vi "Has Run Once.vi"(8 "error in (no error)":errorcluster, 11 "CommandDirector in":refnum<class "CommandDirector.lvclass">) -> (0 "error out":errorcluster, 2 "Has Run Once":bool, 3 "CommandDirector out":refnum<class "CommandDirector.lvclass">)   [LabVIEW 2023, in "HAF.lvlib" / "CommandDirector.lvclass"]
uses:
  CommandDirector.lvclass
  CommandDirector.lvclass/CommandDirector.ctl
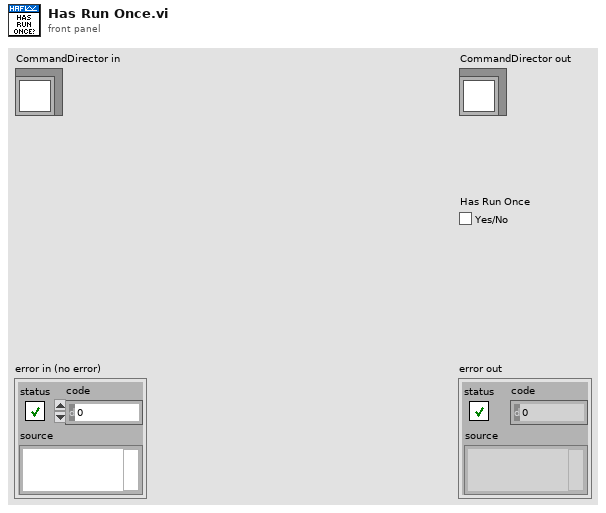
[diagram p1: front panel]
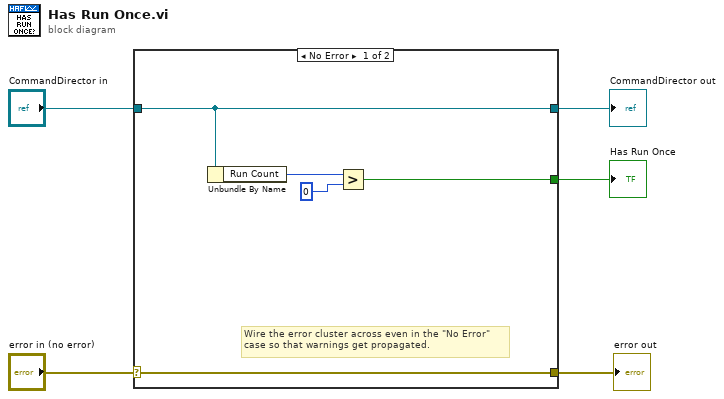
[diagram p0: block diagram]
diagram:
  n1 = case shown="No Error" "error in (no error)" {
    selector: "error in (no error)" -> [w10 w12]
    tunnel: [w10 w12] -> w4
    tunnel: [w6 w11] -> w2
    tunnel: "CommandDirector in" -> [w6 w11]
    tunnel: [w7 _] -> w1
    frame No Error {
      # "Wire the error cluster across even in the \"No Error\"\ncase so that warnings get propagated."
      n2 = Unbundle By Name(w6) -> ("Run Count"=w9:u32)
      n3 = Greater?(x=w9, y=u32 0) -> (0:w7:bool)
    }
    frame Error {
    }
  }
  "error out" <- w4
  "CommandDirector out" <- w2
  "Has Run Once" <- w1
